vi "Agilent SNA Set Smoothing Factor.vi"(6 "Channel":i8=1 min=1 max=99 step=1, 7 "Agilent SNA":T1, 8 "error in (no error)":errorcluster, 10 "Smoothing Factor (%)":dbl, 11 "VISA Resource Names":T2) -> (0 "error out":errorcluster, 3 "dup VISA Resource Names":T2)   [LabVIEW 2011]
doc: "This vi sets the power range. Only works on the HP 8753D."
uses:
  TypeDefs/Agilent SNA VISA.ctl
  TypeDefs/Agilent SNA Instrument Info.ctl
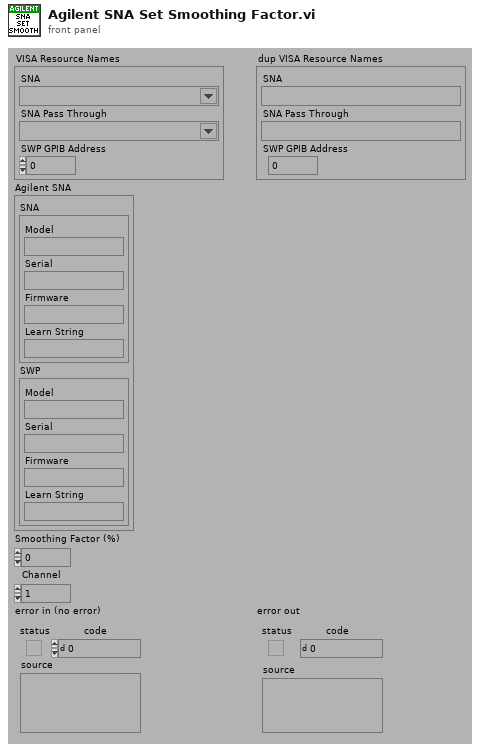
[diagram p1: front panel]
types:
  T1 = typedef "Agilent SNA Instrument Info.ctl" = cluster{"SNA":cluster{"Model":string, "Serial":string, "Firmware":string, "Learn String":string}, "SWP":cluster{"Model":string, "Serial":string, "Firmware":string, "Learn String":string}}
  T2 = typedef "Agilent SNA VISA.ctl" = cluster{"SNA":refnum<visa-resource-name>, "SNA Pass Through":refnum<visa-resource-name>, "SWP GPIB Address":i32}
  T3 = typedef "Agilent SNA Model.ctl" = enum16{"Not Supported", "8757X"}
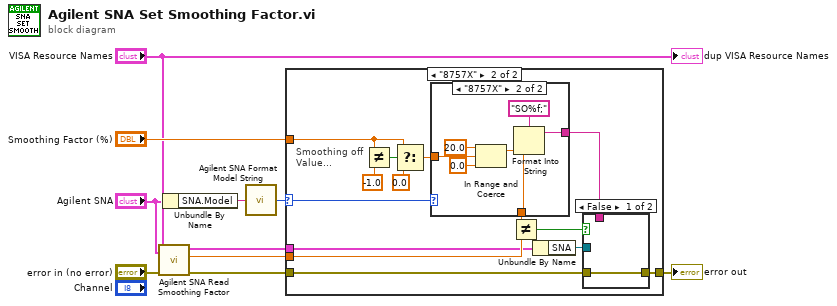
[diagram p0: block diagram]
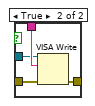
[diagram p4: hidden frame]
diagram:
  n1 = call "Agilent SNA Read Smoothing Factor.vi"("Agilent SNA"="Agilent SNA", "error in (no error)"="error in (no error)", "VISA Resource Names"="VISA Resource Names") -> ("error out"=w8:errorcluster, "Smoothing Factor (%)"=w7:dbl, "dup VISA Resource Names"=w2:T2)  [unwired: 1 in, 5 out]
  n2 = Unbundle By Name("Agilent SNA") -> ("SNA.Model"=w4:string)
  n3 = call "Agilent SNA Format Model String.vi"("Model String"=w4) -> ("Model"=w5:T3)
  n4 = case shown="\"8757X\"" w5 {
    selector: w5 -> [_ w15]
    tunnel: [w11 w25] -> w10
    tunnel: w8 -> [w11 w23]
    tunnel: w2 -> [_ w13]
    tunnel: w7 -> [_ w22]
    tunnel: "Smoothing Factor (%)" -> [_ w17]
    frame "Not Supported" {
    }
    frame "8757X" {
      # "Smoothing off \nValue..."
      n5 = Not Equal?(x=w17, y=-1.0) -> (x != y?=w18:bool)
      n6 = Select(t=w17, s=w18, f=0.0) -> (s? t:f=w16:dbl)
      n7 = case shown="\"8757X\"" w15 {
        tunnel: [_ w30] -> w14
        tunnel: w16 -> [_ w28]
        tunnel: [_ w29] -> w20
        frame "Not Supported" {
        }
        frame "8757X" {
          n8 = In Range and Coerce(upper limit=20.0, x=w28, lower limit=0.0) -> (coerced(x)=w29:dbl)  [unwired: 1 out]
          n9 = Format Into String(format string="SO%f;", w29) -> (resulting string=w30:string)  [unwired: 2 in, 1 out]
        }
      }
      n10 = Not Equal?(x=w20, y=w22) -> (x != y?=w21:bool)
      n11 = Unbundle By Name(w13) -> ("SNA"=w12:refnum<visa-resource-name>)
      n12 = case shown="False" w21 {
        tunnel: [w32 w36] -> w25
        tunnel: w14 -> [_ w35]
        tunnel: w23 -> [w32 w33]
        tunnel: w12 -> [_ w34]
        frame False {
        }
        frame True {
          n13 = VISA Write(VISA resource name=w34, write buffer=w35, error in (no error)=w33) -> (error out=w36:errorcluster)  [unwired: 2 out]
        }
      }
    }
  }
  "error out" <- w10
  "dup VISA Resource Names" <- "VISA Resource Names"
